vi "Translate_XMLHandling - BuildPostData.vi"(9 "TargetLang":T1, 10 "Input text":string, 11 "DeepL authKey":string) -> (3 "String":string)   [LabVIEW 2015, in "lv-deepl-api.lvlib"]
uses:
  lv-deepl-api.lvlib
  TargetLang.ctl
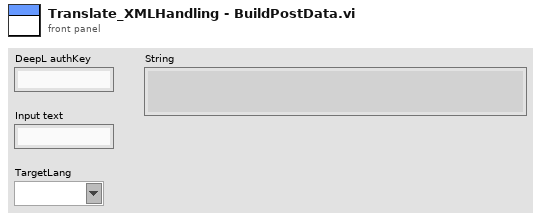
[diagram p1: front panel]
types:
  T1 = typedef "lv-deepl-api.lvlib/TargetLang.ctl" = string
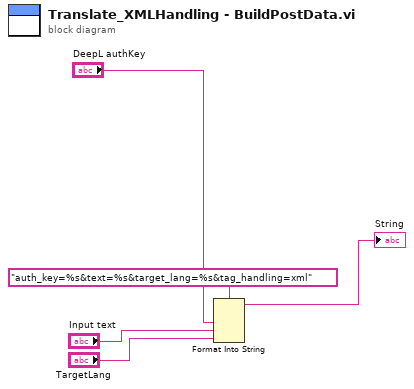
[diagram p0: block diagram]
diagram:
  n1 = Format Into String(format string="auth_key=%s&text=%s&target_lang=%s&tag_handling=xml" ("url"), "DeepL authKey", "Input text", "TargetLang") -> (resulting string=→"String":string)  [unwired: 2 in, 1 out]
